vi "Preserve Volatile State.vi"(7 "Operation":enum16{"Read", "Write", "Update From Data"}(ring), 8 "error in (no error)":errorcluster, 9 "Container State":T2, 10 "Waveform":T1, 11 "Waveform State In":T3={"Measure ?"=[], "Direction"=[], "Loop ?"={"Start"=1, "Finish"=0}, "Storage Location"=[], "Show Current Location"=FALSE, "Current Location"=0, "Show y=0"=FALSE, "Program"=[], "Index"=0, "Average During Loop ?"=FALSE, "# of Loops"=1, "Loop Control"={0, 2}, "Units"="", "Digits"=0, "Significant Figures (F) or DP (T)"=FALSE, "Rate Mode"=FALSE, "Current Y value"=0.0} caption="State" {"# of Loops" min=1 step=1; "Index" min=0 step=1; "Program"."Step" min=0.001 max=80.0 step=0.001 format="%.2f"; "Program"."Target" format="%.2f"}) -> (0 "error out":errorcluster, 2 "Waveform Out":T1, 3 "Waveform State Out":T3={"Measure ?"=[], "Direction"=[], "Loop ?"={"Start"=1, "Finish"=0}, "Storage Location"=[], "Show Current Location"=FALSE, "Current Location"=0, "Show y=0"=FALSE, "Program"=[], "Index"=0, "Average During Loop ?"=FALSE, "# of Loops"=1, "Loop Control"={0, 2}, "Units"="", "Digits"=0, "Significant Figures (F) or DP (T)"=FALSE, "Rate Mode"=FALSE, "Current Y value"=0.0} caption="State" {"# of Loops" min=1 step=1; "Index" min=0 step=1; "Program"."Step" min=0.001 max=80.0 step=0.001 format="%.2f"; "Program"."Target" format="%.2f"})   [LabVIEW 2012, in "Multi Segment Waveform.xctl"]
doc: "Saves the XControl state to a LV2 style global thathandles multiple instances of the control"
uses:
  Multi Segment Waveform.xctl
  State.ctl
  <vilib>/_xctls/Container State.ctl
  Data.ctl
  <vilib>/_xctls/XControlSupport.lvlib
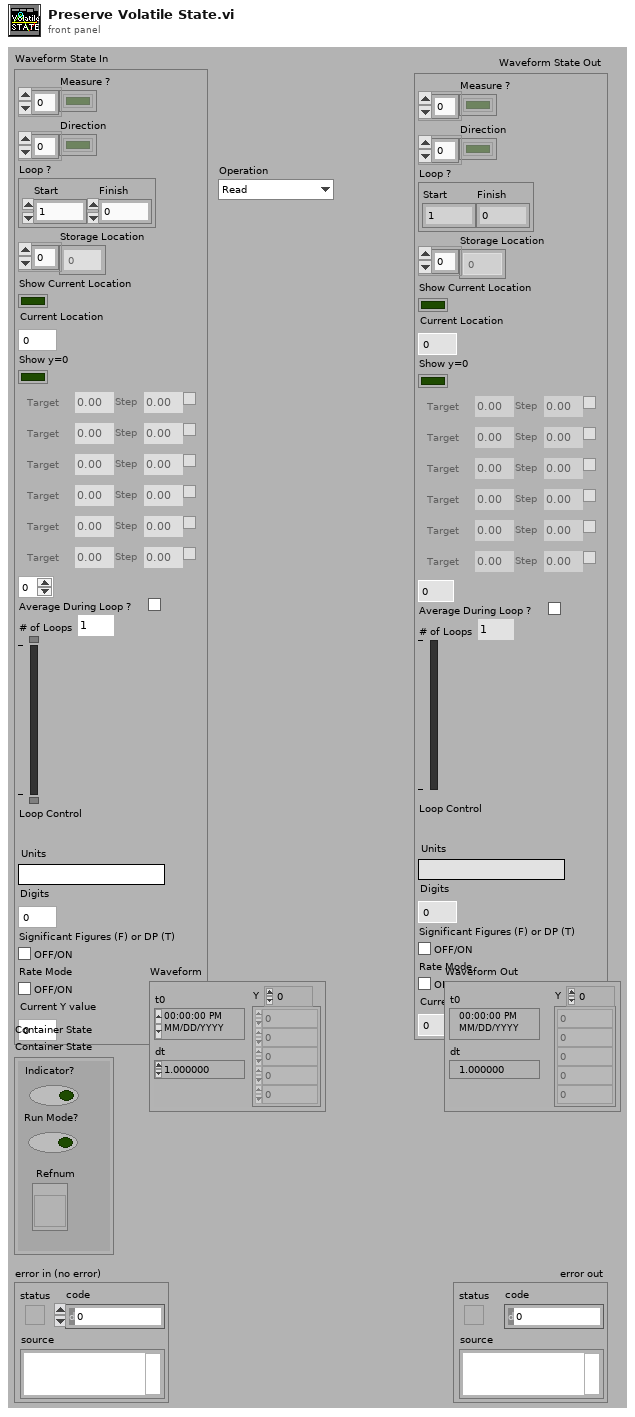
[diagram p1: front panel]
types:
  T1 = typedef "Multi Segment Waveform.xctl/Data.ctl" = waveform(dbl)
  T2 = typedef "XControlSupport.lvlib/Container State.ctl" = cluster{"Indicator?":bool, "Run Mode?":bool, " Refnum":refnum<vi>}
  T3 = typedef "Multi Segment Waveform.xctl/State.ctl" = cluster{"Measure ?":bool[], "Direction":bool[], "Loop ?":cluster{"Start":i32, "Finish":i32}, "Storage Location":i32[], "Show Current Location":bool, "Current Location":i32, "Show y=0":bool, "Program":cluster{"Target":dbl, "Step":dbl, "Measure ?":bool}[], "Index":i32, "Average During Loop ?":bool, "# of Loops":u32, "Loop Control":cluster{i32, i32}, "Units":string, "Digits":i32, "Significant Figures (F) or DP (T)":bool, "Rate Mode":bool, "Current Y value":dbl}
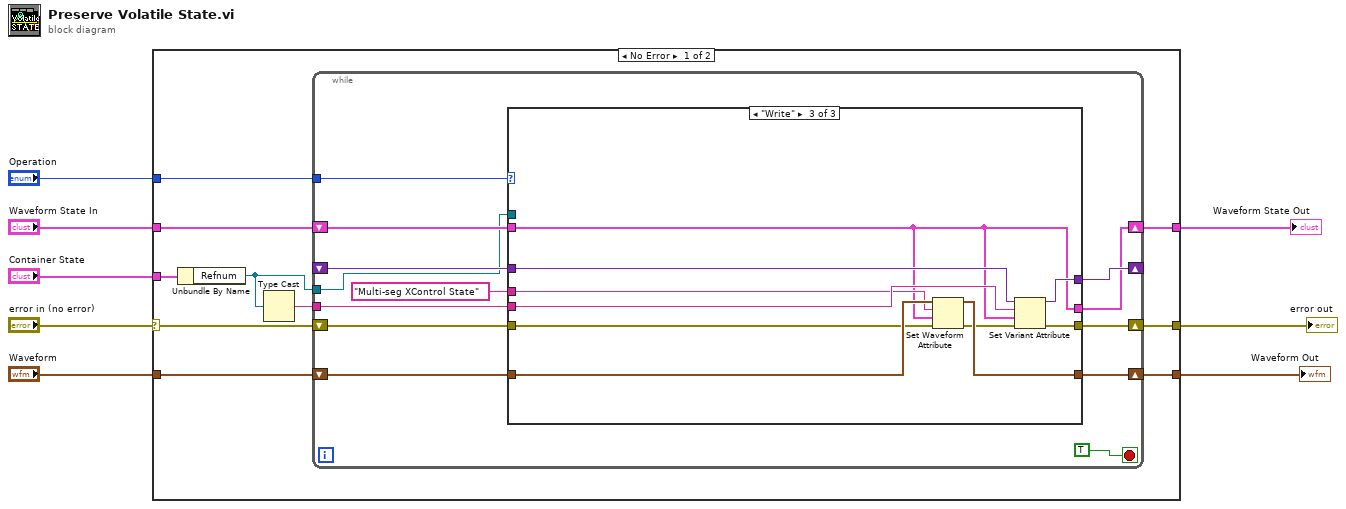
[diagram p0: block diagram]
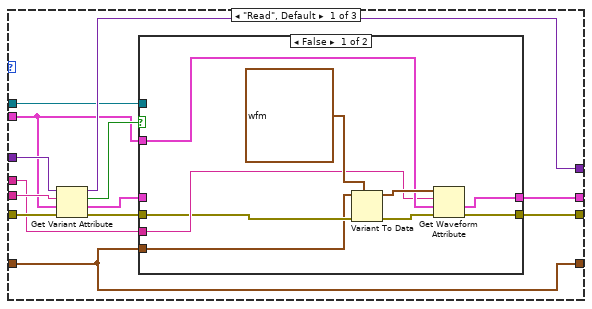
[diagram p2: hidden frame]
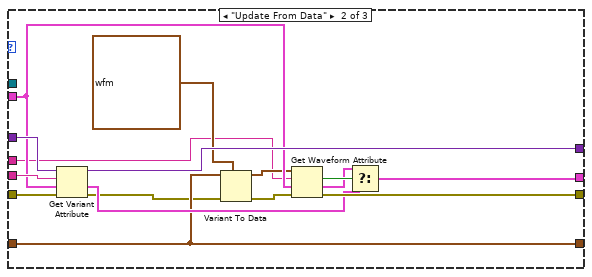
[diagram p4: hidden frame]
diagram:
  n1 = case shown="No Error" "error in (no error)" {
    selector: "error in (no error)" -> [w13 w84]
    tunnel: "Container State" -> [w18 _]
    tunnel: "Operation" -> [w16 _]
    tunnel: "Waveform State In" -> [w15 w83]
    tunnel: [w12 w84] -> w4
    tunnel: [w11 w83] -> w3
    tunnel: "Waveform" -> [w10 w82]
    tunnel: [w9 w82] -> w1
    frame No Error {
      n2 = Unbundle By Name(w18) -> ("Refnum"=w14:refnum<vi>)
      n3 = Type Cast(x=w14) -> (*(type *) &x=w17:string)  [unwired: 1 out]
      n4 = while {
        shift-right: [w30] -> _
        shift-left: _ -> [w31]
        tunnel: w17 -> [w27]
        tunnel: w16 -> [w29]
        tunnel: w14 -> [w26]
        shift-right: [w24] -> w12
        shift-left: w13 -> [w25]
        shift-right: [w23] -> w11
        shift-left: w15 -> [w28]
        shift-right: [w20] -> w9
        shift-left: w10 -> [w19]
        stop <- TRUE stop-if-true
        n5 = case shown="\"Write\"" w29 {
          tunnel: w31 -> [w44 w71 w81]
          tunnel: [w43 w70 w80] -> w30
          tunnel: w28 -> [w37 w67 w72]
          tunnel: w27 -> [w42 w69 w79]
          tunnel: w26 -> [w40 _ _]
          tunnel: w25 -> [w39 w68 w74]
          tunnel: [w36 w66 w78] -> w24
          tunnel: [w35 w59 w72] -> w23
          tunnel: "Multi-seg XControl State" ("name") -> [w33 w58 w75]
          tunnel: [w32 w57 w76] -> w20
          tunnel: w19 -> [w32 w57 w77]
          frame "Read", Default {
            n6 = Get Variant Attribute(Variant=w44, name=w42, default value (empty Variant)=w37, error in=w39) -> (duplicate Variant=w43:variant, found=w41:bool, value=w34:T3, error out=w38:errorcluster)
            n7 = case shown="False" w41 {
              tunnel: w40 -> [_ _]
              tunnel: w38 -> [w46 w55]
              tunnel: w37 -> [w50 _]
              tunnel: [w49 w54] -> w35
              tunnel: [w48 w55] -> w36
              tunnel: w34 -> [_ w54]
              tunnel: w33 -> [w47 _]
              tunnel: w32 -> [w45 _]
              frame False {
                n8 = Variant To Data(error in=w46, type=waveform(dbl) {"t0"=timestamp(0 s since 1904-01-01), "dt"=1.0, "Y"=[]} ("waveform"), Variant=w45) -> (data=w52:waveform(dbl), error out=w51:errorcluster)
                n9 = Get Waveform Attribute(4:w51, 5:w50, 6:w47, 7:w52) -> (0:w48:errorcluster, 1:w49:T3)  [unwired: 2 out]
              }
              frame True {
              }
            }
          }
          frame "Update From Data" {
            n10 = Get Variant Attribute(Variant=w71, name=w69, default value (empty Variant)=w67, error in=w68) -> (duplicate Variant=w70:variant, value=w60:T3, error out=w56:errorcluster)  [unwired: 1 out]
            n11 = Variant To Data(error in=w56, type=waveform(dbl) {"t0"=timestamp(0 s since 1904-01-01), "dt"=1.0, "Y"=[]} ("waveform"), Variant=w57) -> (data=w64:waveform(dbl), error out=w63:errorcluster)
            n12 = Get Waveform Attribute(4:w63, 5:w67, 6:w58, 7:w64) -> (0:w66:errorcluster, 1:w61:T3, 2:w62:bool)  [unwired: 1 out]
            n13 = Select(t=w61, s=w62, f=w60) -> (s? t:f=w59:T3)
          }
          frame "Write" {
            n14 = Set Waveform Attribute(4:w74, 5:w72, 6:w75, 7:w77) -> (0:w73:errorcluster, 3:w76:T1)  [unwired: 1 out]
            n15 = Set Variant Attribute(Variant=w81, name=w79, value=w72, error in=w73) -> (Variant out=w80:variant, error out=w78:errorcluster)  [unwired: 1 out]
          }
        }
      }
    }
    frame Error {
    }
  }
  "error out" <- w4
  "Waveform State Out" <- w3
  "Waveform Out" <- w1
